vi "Add dev dist if present.vi"(11 "paths in":path[](array[path])) -> (3 "paths out":path[](array[path]))   [LabVIEW 2020]
doc: "Dev builds of LabVIEW keep the majority of their files in a separate directory from the executable. If this directory exists, include it in LibraryPaths."
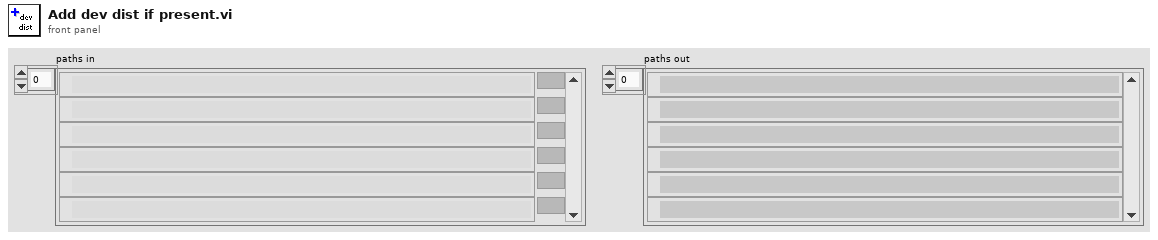
[diagram p1: front panel]
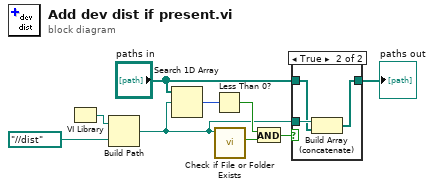
[diagram p0: block diagram]
diagram:
  n1 = VI Library() -> (path=w9:path)
  n2 = Build Path(base path=w9, name or relative path=path "../../dist") -> (appended path=w3:path)
  n3 = Search 1D Array(1D array="paths in", element=w3) -> (index of element=w7:i32)  [unwired: 1 in]
  n4 = Less Than 0?(x=w7) -> (x < 0?=w5:bool)
  n5 = call <vilib>:"Check if File or Folder Exists.vi"("path"=w3) -> ("file or folder exists?"=w6:bool)  [unwired: 8 in, 2 out]
  n6 = And(x=w5, y=w6) -> (x .and. y?=w4:bool)
  n7 = case shown="True" w4 {
    tunnel: w3 -> [_ w13]
    tunnel: "paths in" -> [w10 w12]
    tunnel: [w10 w11] -> w1
    frame False {
    }
    frame True {
      n8 = Build Array (concatenate)(w13, w12) -> (w11:path[])
    }
  }
  "paths out" <- w1
